vi "Redline Data.vi"(7 "Aborts in":bool[](array[boolean]), 10 "Data":dbl[][](array[numeric]), 11 "Params":dbl[][](array[numeric])) -> (2 "Scaled Data":dbl[][](array[numeric]), 5 "Aborts":bool[](array[boolean]))   [LabVIEW 2020]
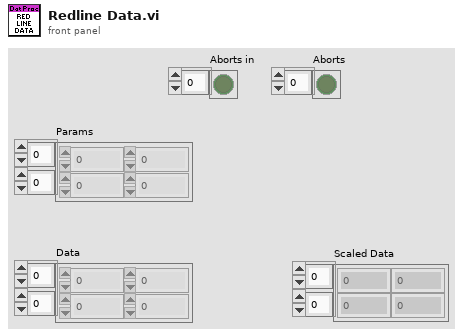
[diagram p1: front panel]
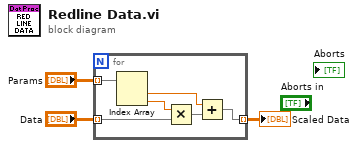
[diagram p0: block diagram]
diagram:
  n1 = for {
    tunnel: "Params" -> [w9] mode=indexing
    tunnel: "Data" -> [w8] mode=indexing
    tunnel: [w4] -> w1 mode=indexing
    n2 = Index Array(array=w9) -> (element #1=w5:dbl, element #2=w7:dbl)  [unwired: 2 in]
    n3 = Multiply(x=w7, y=w8) -> (x*y=w6:dbl[])
    n4 = Add(x=w5, y=w6) -> (x+y=w4:dbl[])
  }
  "Scaled Data" <- w1
